vi "Test Explorer.vi"() -> ()   [LabVIEW 2017, in "Test Explorer.lvlib"]
uses:
  Test Explorer.lvlib
  Test Case/Test Case.lvclass
  Test Result/Test Result.lvclass
  LVUnit Test Discoverer/LVUnit Test Discoverer.lvclass
  Test Case/Test Case.lvclass/Test Case.ctl
  LVUnit Test Executor/LVUnit Test Executor.lvclass
  Test Outcome.ctl
  Test Result/Test Result.lvclass/Test Result.ctl
  <vilib>/Utility/sysdir.llb/System Directory Type.ctl
  Test Case/Get Qualified Name.vi
  Test Result/Get Outcome.vi
  ResultTree/ResultTree.lvclass
panel:
  in  "Export...":bool
  out "#Not Executed":i32
  out "#Total":i32
  out "#Failed":i32
  out "#Passed":i32
  out "Timer":dbl format="%<%H:%M:%S%3u>t"
  in  "Run All":bool
  in  "Result Tree":string(tree)
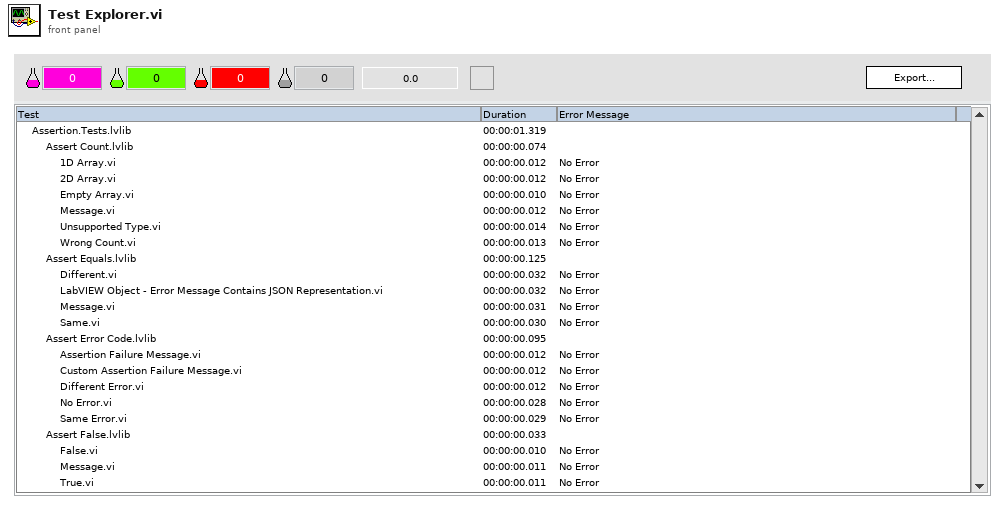
[diagram p1: front panel]
types:
  T1 = typedef "Test Outcome.ctl" = enum16{"None", "Passed", "Failed"}
  T2 = typedef "System Directory Type.ctl" = i32
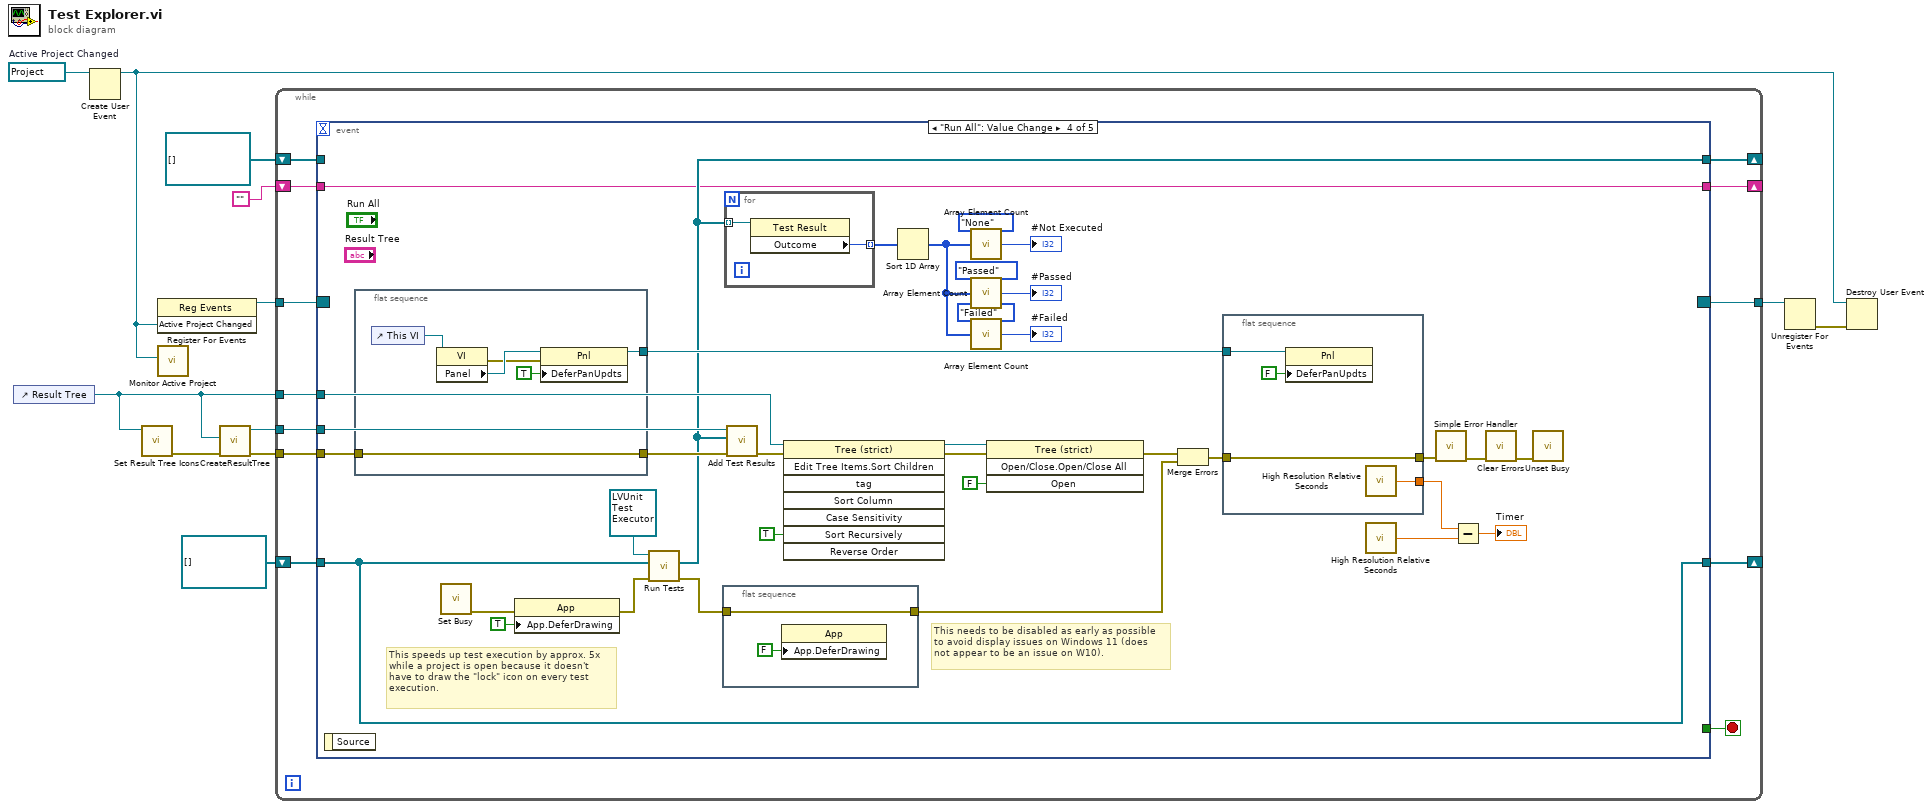
[diagram p0: block diagram]
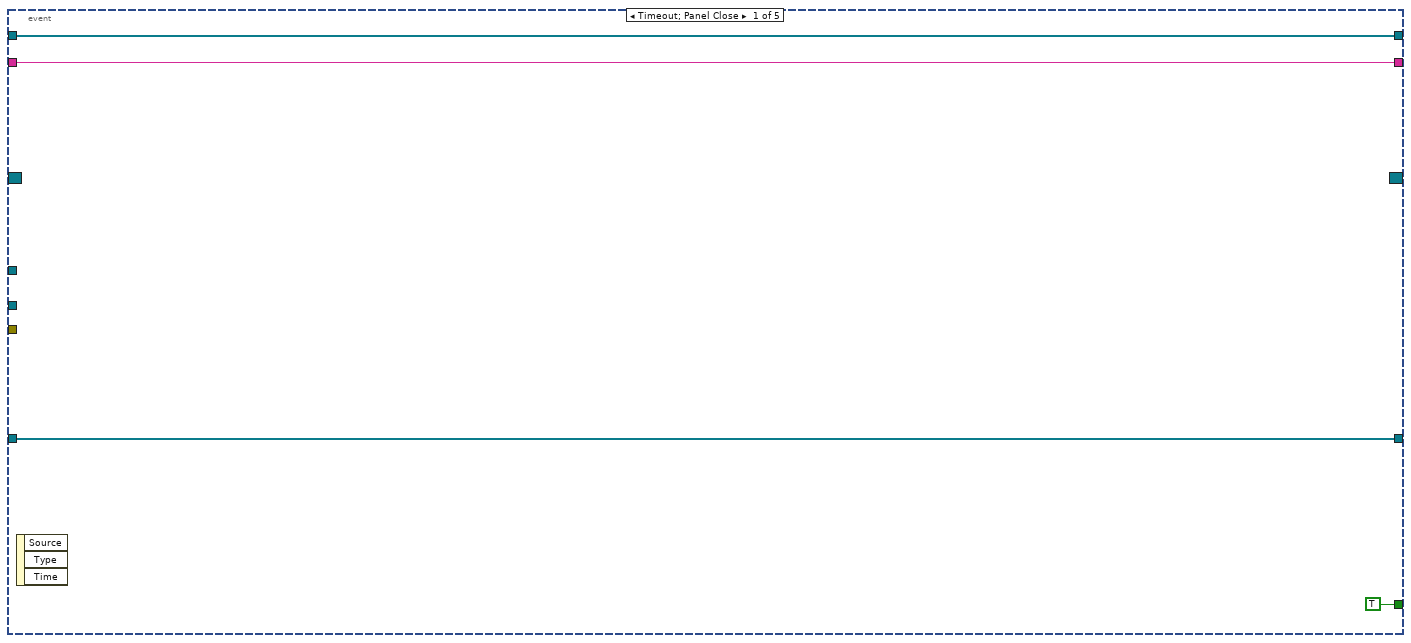
[diagram p2: hidden frame]
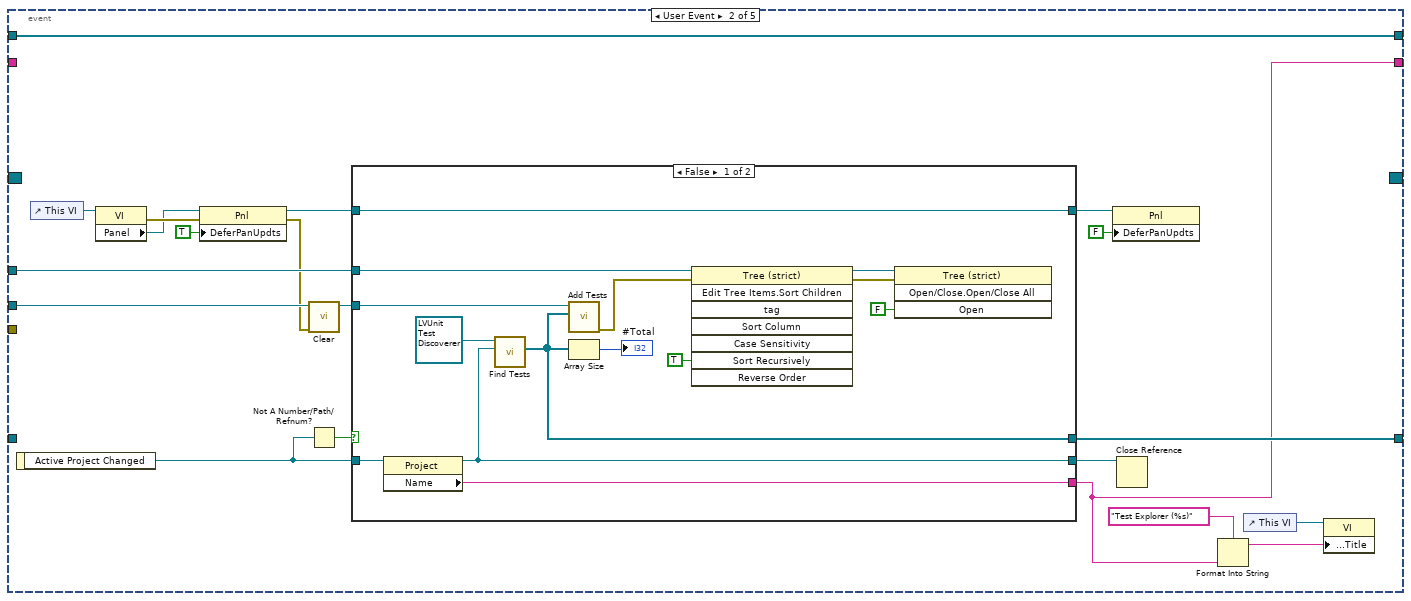
[diagram p3: hidden frame]
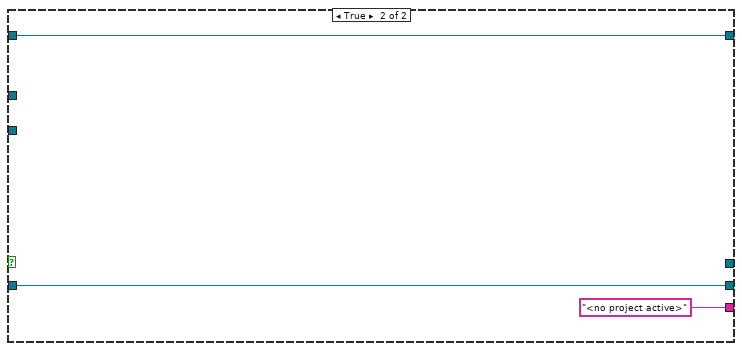
[diagram p4: hidden frame]
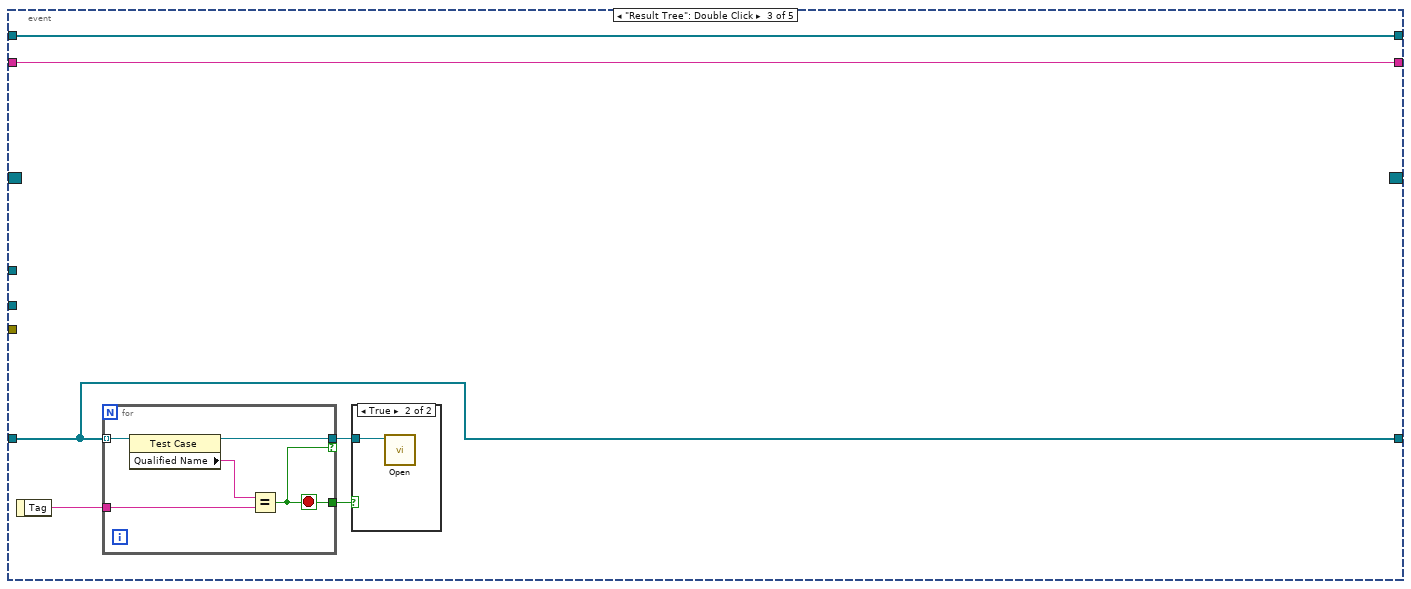
[diagram p5: hidden frame]
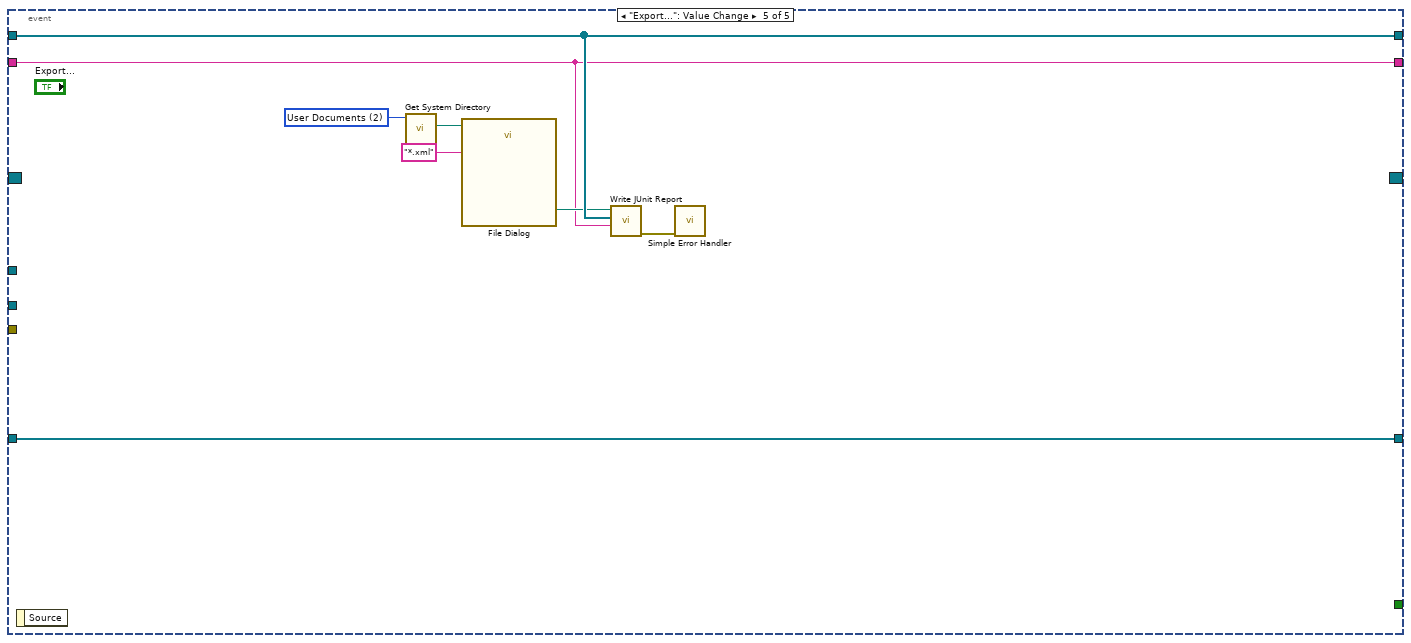
[diagram p7: hidden frame]
diagram:
  w8 = refnum<vi> refnum  # Active Project Changed
  n1 = control-ref of="Result Tree"() -> (w10:refnum<vi>)
  n2 = Create User Event(user event datatype=w8) -> (user event=w4:refnum<user-event>)  [unwired: 1 in, 1 out]
  n3 = call "Set Result Tree Icons.vi"("Tree Refnum"=w10) -> ("error out"=w12:errorcluster)  [unwired: 10 in]
  n4 = register-events(w4) -> (reference out=w7:refnum<event-registration>)  [unwired: 2 in, 1 out]
  n5 = call "Monitor Active Project.vi"("Active Project Changed"=w4) -> ()  [unwired: 11 in]
  n6 = call "CreateResultTree.vi"("error in (no error)"=w12, "Tree Refnum"=w10) -> ("error out"=w11:errorcluster, "ResultTree out"=w9:refnum<class "ResultTree.lvclass">)  [unwired: 8 in]
  n7 = while {
    tunnel: w10 -> [w23]
    tunnel: w11 -> [w22]
    tunnel: w9 -> [w21]
    tunnel: w7 -> [w20]
    tunnel: [w19] -> w6
    shift-right: [w18] -> _
    shift-left: refnum<class "Test Case.lvclass">[] [] ("Test Cases") -> [w17]
    shift-right: [w16] -> _
    shift-left: refnum<class "Test Result.lvclass">[] [] ("Test Results") -> [w15]
    shift-right: [w14] -> _
    shift-left: "" -> [w13]
    stop <- w24 stop-if-true
    n8 = event shown="[3] \"Run All\": Value Change" {
      selector: w20 -> [_ _ _ _ _]
      dyn-events: [_ _ _ _ _] -> w19
      timeout: _ -> [_ _ _ _ _]
      tunnel: [TRUE _ _ _ _] -> w24
      tunnel: w23 -> [_ w44 _ w106 _]
      tunnel: w22 -> [_ _ _ w81 _]
      tunnel: w21 -> [_ w46 _ w105 _]
      tunnel: [w27 w35 w68 w103 w134] -> w18
      tunnel: w17 -> [w27 _ w68 w103 w134]
      tunnel: [w26 w30 w67 w79 w132] -> w16
      tunnel: w15 -> [w26 w30 w67 _ w132]
      tunnel: [w25 w29 w66 w78 w127] -> w14
      tunnel: w13 -> [w25 _ w66 w78 w127]
      event Timeout; Panel Close {
        n9 = event-data() -> ()  [unwired: 1 in, 3 out]
      }
      event User Event {
        n10 = event-data() -> ("Active Project Changed"=w48:refnum<vi>)  [unwired: 1 in]
        n11 = control-ref of="This VI"() -> (w41:refnum<vi>)
        n12 = property class="VI"(reference=w41) -> (error out=w43:errorcluster, "Panel"=w42:refnum<vi>)  [unwired: 1 in, 1 out]
        n13 = property class="Pnl"(reference=w42, error in=w43, "DeferPanUpdts"=TRUE ("Defer Panel Updates")) -> (reference out=w39:refnum<vi>, error out=w36:errorcluster)
        n14 = call "Clear.vi"("error in (no error)"=w36, "ResultTree in"=w46) -> ("ResultTree out"=w45:refnum<class "ResultTree.lvclass">)  [unwired: 8 in, 1 out]
        n15 = Not A Number/Path/Refnum?(number/path/refnum=w48) -> (NaN/Path/Refnum?=w47:bool)
        n16 = case shown="False" w47 {
          tunnel: w48 -> [w62 w63]
          tunnel: [w61 "<no project active>" ("Name")] -> w29
          tunnel: w45 -> [w59 _]
          tunnel: w44 -> [w54 _]
          tunnel: w39 -> [w52 w64]
          tunnel: [w52 w64] -> w37
          tunnel: [w51 _] -> w35
          tunnel: [w50 w63] -> w34
          frame False {
            n17 = property class="Project"(reference=w62) -> (reference out=w50:refnum<vi>, "Name"=w61:string)  [unwired: 1 in, 1 out]
            n18 = call-dynamic "Find Tests.vi"("Project Refnum"=w50, "LVUnit Test Discoverer in"=refnum<class "LVUnit Test Discoverer.lvclass"> refnum ("LVUnit Test Discoverer")) -> ("Test Cases"=w51:refnum<class "Test Case.lvclass">[])  [unwired: 7 in, 2 out]
            n19 = call "Add Tests.vi"("Test Cases"=w51, "ResultTree in"=w59) -> ("error out"=w53:errorcluster)  [unwired: 8 in, 1 out]
            n20 = Array Size(array=w51) -> (size(s)=→"#Total":i32)
            n21 = invoke class="Tree (strict)" method="Edit Tree Items.Sort Children"(reference=w54, error in=w53, "Sort Recursively"=TRUE ("Sort Recursively?")) -> (reference out=w58:refnum<vi>, error out=w57:errorcluster)  [unwired: 5 in, 6 out]
            n22 = invoke class="Tree (strict)" method="Open/Close.Open/Close All"(reference=w58, error in=w57, "Open"=FALSE ("Open?")) -> ()  [unwired: 1 in, 4 out]
          }
          frame True {
          }
        }
        n23 = property class="Pnl"(reference=w37, "DeferPanUpdts"=FALSE ("Defer Panel Updates")) -> ()  [unwired: 1 in, 2 out]
        n24 = Close Reference(reference=w34) -> ()  [unwired: 1 in, 1 out]
        n25 = Format Into String(format string="Test Explorer (%s)" ("string"), w29) -> (resulting string=w31:string)  [unwired: 2 in, 1 out]
        n26 = control-ref of="This VI"() -> (w33:refnum<vi>)
        n27 = property class="VI"(reference=w33, "Front Panel.Title"=w31) -> ()  [unwired: 1 in, 2 out]
      }
      event "Result Tree": Double Click {
        n28 = event-data() -> ("Tag"=w71:string)  [unwired: 1 in]
        n29 = for {
          tunnel: w68 -> [w77] mode=indexing
          tunnel: w71 -> [w76]
          tunnel: [w74] -> w70 if=w73
          tunnel: [w73] -> w69
          stop <- w73 stop-if-true
          n30 = property class="Test Case"(reference=w77) -> (reference out=w74:refnum<class "Test Case.lvclass">, "Qualified Name"=w75:string)  [unwired: 1 in, 1 out]
          n31 = Equal?(x=w75, y=w76) -> (x = y?=w73:bool)
        }
        n32 = case shown="True" w69 {
          tunnel: w70 -> [_ w72]
          frame False {
          }
          frame True {
            n33 = call-dynamic "Open.vi"("Test Case in"=w72) -> ()  [unwired: 9 in, 2 out]
          }
        }
      }
      event "Run All": Value Change {
        # "This needs to be disabled as early as possible\nto avoid display issues on Windows 11 (does\nnot appear to be an issue on W10)."
        # "This speeds up test execution by approx. 5x\nwhile a project is open because it doesn't\nhave to draw the \"lock\" icon on every test\nexecution."
        n34 = event-data() -> ()  [unwired: 1 in, 1 out]
        n35 = flat-sequence {
          tunnel: [w114] -> w82
          tunnel: w81 -> [w113]
          tunnel: [w113] -> w80
          frame #0 {
            n36 = control-ref of="This VI"() -> (w118:refnum<vi>)
            n37 = property class="VI"(reference=w118) -> (error out=w116:errorcluster, "Panel"=w117:refnum<vi>)  [unwired: 1 in, 1 out]
            n38 = property class="Pnl"(reference=w117, error in=w116, "DeferPanUpdts"=TRUE ("Defer Panel Updates")) -> (reference out=w114:refnum<vi>)  [unwired: 1 out]
          }
        }
        n39 = call <vilib>:"Set Busy.vi"() -> ("error out"=w104:errorcluster)  [unwired: 10 in, 1 out]
        n40 = property class="App"(error in=w104, "App.DeferDrawing"=TRUE ("Application:Defer Drawing")) -> (error out=w97:errorcluster)  [unwired: 1 in, 1 out]
        n41 = call-dynamic "Run Tests.vi"("error in (no error)"=w97, "Test Cases"=w103, "LVUnit Test Executor in"=refnum<class "LVUnit Test Executor.lvclass"> refnum ("LVUnit Test Executor")) -> ("error out"=w83:errorcluster, "Test Results"=w79:refnum<class "Test Result.lvclass">[])  [unwired: 6 in, 1 out]
        n42 = flat-sequence {
          tunnel: [w119] -> w84
          tunnel: w83 -> [w119]
          frame #0 {
            n43 = property class="App"("App.DeferDrawing"=FALSE ("Application:Defer Drawing")) -> ()  [unwired: 2 in, 2 out]
          }
        }
        n44 = for {
          tunnel: w79 -> [w122] mode=indexing
          tunnel: [w121] -> w92 mode=indexing
          n45 = property class="Test Result"(reference=w122) -> ("Outcome"=w121:T1)  [unwired: 1 in, 2 out]
        }
        n46 = call "Add Test Results.vi"("error in (no error)"=w80, "Test Results"=w79, "ResultTree in"=w105) -> ("error out"=w100:errorcluster)  [unwired: 7 in, 1 out]
        n47 = invoke class="Tree (strict)" method="Edit Tree Items.Sort Children"(reference=w106, error in=w100, "Sort Recursively"=TRUE ("Sort Recursively?")) -> (reference out=w107:refnum<vi>, error out=w108:errorcluster)  [unwired: 5 in, 6 out]
        n48 = Sort 1D Array(array=w92) -> (sorted array=w91:T1[])
        n49 = call "Array Element Count.vi"("Array"=w91, "Element"=Test_Outcome."None" ("Outcome")) -> ("Count"=→"#Not Executed":i16)
        n50 = call "Array Element Count.vi"("Array"=w91, "Element"=Test_Outcome."Passed" ("Outcome")) -> ("Count"=→"#Passed":i16)
        n51 = call "Array Element Count.vi"("Array"=w91, "Element"=Test_Outcome."Failed" ("Outcome")) -> ("Count"=→"#Failed":i16)
        n52 = invoke class="Tree (strict)" method="Open/Close.Open/Close All"(reference=w107, error in=w108, "Open"=FALSE ("Open?")) -> (error out=w101:errorcluster)  [unwired: 1 in, 3 out]
        n53 = Merge Errors(w101, w84) -> (w98:errorcluster)
        n54 = flat-sequence {
          tunnel: w98 -> [w126]
          tunnel: [w126] -> w99
          tunnel: [w125] -> w96
          tunnel: w82 -> [w123]
          frame #0 {
            n55 = property class="Pnl"(reference=w123, "DeferPanUpdts"=FALSE ("Defer Panel Updates")) -> ()  [unwired: 1 in, 2 out]
            n56 = call <vilib>:"High Resolution Relative Seconds.vi"() -> ("relative seconds"=w125:dbl)
          }
        }
        n57 = call <vilib>:"High Resolution Relative Seconds.vi"() -> ("relative seconds"=w95:dbl)
        n58 = call <vilib>:"Simple Error Handler.vi"("error in (no error)"=w99) -> ("error out"=w111:errorcluster)  [unwired: 4 in, 4 out]
        n59 = Subtract(x=w96, y=w95) -> (x-y=→"Timer":dbl)
        n60 = call <vilib>:"Clear Errors.vi"("error in (no error)"=w111) -> ("error out"=w112:errorcluster)  [unwired: 5 in, 1 out]
        n61 = call <vilib>:"Unset Busy.vi"("error in (no error)"=w112) -> ()  [unwired: 10 in, 1 out]
      }
      event "Export...": Value Change {
        w129 = T2 2 items=["User Home"=0, "User Desktop"=1, "User Documents"=2, "User Application Data"=3, "User Preferences"=4, "User Temporary"=5, "Public Documents"=6, "Public Application Data"=7, "Public Preferences"=8, "Public Cache"=13, "System Core Libraries"=9, "System Installed Libraries"=10, "Application Files"=11, "Boot Volume Root"=12] ("system directory type")
        n62 = event-data() -> ()  [unwired: 1 in, 1 out]
        n63 = call <vilib>:"Get System Directory.vi"("system directory type"=w129) -> ("system directory"=w130:path)  [unwired: 10 in]
        n64 = call "File Dialog"("start path"=w130, "pattern (all files)"="*.xml") -> ("selected path"=w131:path)  [unwired: 10 in, 3 out]
        n65 = call "Write JUnit Report.vi"("Project Name"=w127, "Test Results"=w132, "File Path"=w131) -> ("error out"=w133:errorcluster)  [unwired: 8 in]
        n66 = call <vilib>:"Simple Error Handler.vi"("error in (no error)"=w133) -> ()  [unwired: 4 in, 5 out]
      }
    }
  }
  n67 = Unregister For Events(event registration refnum=w6) -> (error out=w5:errorcluster)  [unwired: 1 in]
  n68 = Destroy User Event(user event=w4, error in=w5) -> ()  [unwired: 1 out]
